vi "INI.vi"(0 "System no.":i32=1 min=1 max=4 step=1, 2 "INI axes":string[](array[string]), 3 "All axes?":bool, 4 "Axis identifier?":bool=TRUE, 5 "error in":errorcluster) -> (19 "error out":errorcluster)   [LabVIEW 2020]
doc: "Initializes axes. System-specific: see individual GCS-DLL or system manual for details.\n\nC-702: If All axes = TRUE, then Axis identifier must be TRUE\n\nC-843: If All axes = TRUE, then Axis identifier must be TRUE\n\nC-843.PM: If All axes = TRUE, then Axis identifier must be TRUE\n\nC-844: If All axes = TRUE, then Axis identifier must be TRUE, It is necessary to wait a certain time - appr. 4 s - before sending the next command to prevent it from being lost.\n\nC-848: If All axes = TRUE, then Axis identifier must be TRUE\n\nC-865: If All axes = TRUE, then Axis identifier must be TRUE\n\nC-866: If All axes? = TRUE, then Axis identifier? must be TRUE\n\nC-880: If All axes = TRUE, then Axis identifier must be TRUE\n\nC-885: All axes must beTRUE, Axis identifier must be FALSE\n\nE-710: If All axes = TRUE, then Axis identifier must be TRUE\n\nC-887, F-206, M-8X0: Only for GCS syntax version = GCS 1.0 (Check with CSV?.vi. If CSV?.vi is not supported, syntax version is GCS 1.0). For GCS 2.0 or higher, VI calls FRF instead for compatibility. To initialize hexapod, All axes = TRUE, Axis identifier = FALSE, (separate axes A,B (if present) will not be initialized); to initialize axes A,B: All axes = FALSE; VI will not wait for INI procedure to finish. Depending on the firmware version on the controller, motion initiated by INI may not be able to be stopped by STOP, #24 or #27.\n\nHydra, Pollux: If All axes? = TRUE, then Axis identifier? can be FALSE.\n\nMercury: If All axes = TRUE, then Axis identifier can be FALSE"
uses:
  Controller names.ctl
  Syntax.ctl
  Global2 (Array).vi
  Global1.vi
panel:
  # "Initializes axes. System-specific: see individual\nGCS-DLL or system manual for details."
  # "If all axes: use"
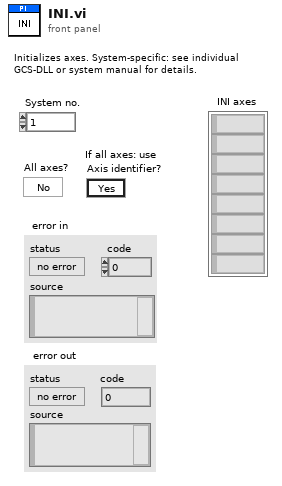
[diagram p1: front panel]
types:
  T1 = typedef "Syntax.ctl" = enum16{"GCS 1.0", "GCS 2.0", "GCS 3.0"}
  T2 = typedef "Controller names.ctl" = enum16{"None", "Analog", "C-702", "C-413", "C-414", "C-843", "C-843.PM", "C-844", "C-848", "C-865", "C-866", "C-867", "C-877", "C-880", "C-884", "C-885", "C-886", "C-887", "C-891", "E-135", "E-516", "E-517", "E-518", "E-709", "E-710", "E-712", "E-725", "E-727", "E-753", "E-754", "E-755", "E-761", "E-816", "E-861", "E-870", "E-871", "E-872", "E-873", "E-874", "F-206", "HydraPollux", "M-840", "M-850", "M-8X0", "Mercury", "Mercury_GCS", "PI_GCS2"}
  T3 = cluster{"Conn. axes":string[], "Controller name":T2}[]
  T4 = cluster{"Conn. axes":string[], "Controller name":T2}
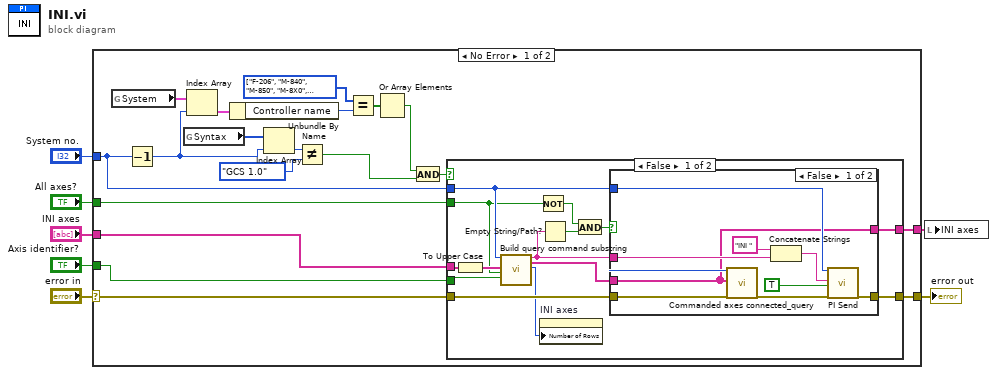
[diagram p0: block diagram]
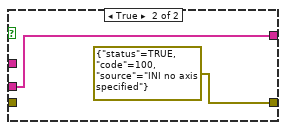
[diagram p2: hidden frame]
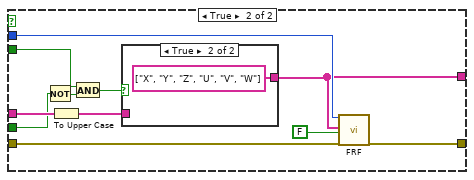
[diagram p3: hidden frame]
diagram:
  n1 = case shown="No Error" "error in" {
    selector: "error in" -> [w11 w66]
    tunnel: "INI axes" -> [w26 w65]
    tunnel: "Axis identifier?" -> [w25 _]
    tunnel: "System no." -> [w13 _]
    tunnel: "All axes?" -> [w24 _]
    tunnel: [w23 w66] -> w3
    tunnel: [w10 w65] -> w1
    frame No Error {
      w21 = T2[] [enum."F-206", enum."M-840", enum."M-850", enum."M-8X0", enum."C-887"] items=["None", "Analog", "C-702", "C-413", "C-414", "C-843", "C-843.PM", "C-844", "C-848", "C-865", "C-866", "C-867", "C-877", "C-880", "C-884", "C-885", "C-886", "C-887", "C-891", "E-135", "E-516", "E-517", "E-518", "E-709", "E-710", "E-712", "E-725", "E-727", "E-753", "E-754", "E-755", "E-761", "E-816", "E-861", "E-870", "E-871", "E-872", "E-873", "E-874", "F-206", "HydraPollux", "M-840", "M-850", "M-8X0", "Mercury", "Mercury_GCS", "PI_GCS2"]
      n2 = global read "Global2 (Array).vi" "System"() -> (w18:T3)
      n3 = Decrement(x=w13) -> (x-1=w9:i32)
      n4 = global read "Global1.vi" "Syntax"() -> (w17:T1[])
      n5 = Index Array(array=w18, index=w9) -> (element=w19:T4)
      n6 = Unbundle By Name(w19) -> ("Controller name"=w20:T2)
      n7 = Index Array(array=w17, index=w9) -> (element=w16:T1)
      n8 = Not Equal?(x=w16, y=Syntax."GCS 1.0") -> (x != y?=w15:bool)
      n9 = Equal?(x=w21, y=w20) -> (x = y?=w22:bool[])
      n10 = Or Array Elements(Boolean array=w22) -> (logical OR=w14:bool)
      n11 = And(x=w14, y=w15) -> (x .and. y?=w12:bool)
      n12 = case shown="False" w12 {
        tunnel: w11 -> [w40 w60]
        tunnel: w26 -> [w39 w62]
        tunnel: w25 -> [w37 w54]
        tunnel: w13 -> [w36 w61]
        tunnel: w24 -> [w34 w55]
        tunnel: [w32 w57] -> w23
        tunnel: [w31 w52] -> w10
        frame False {
          n13 = To Upper Case(1:w39) -> (0:w38:string[])
          n14 = call "Build query command substring.vi"("System no."=w36, "Axes to query in"=w38, "Query\nAll axes?"=w34, "For all axes: use\nAxis identifier?"=w37) -> ("Command substring"=w28:string, "Axes to query out"=w30:string[], "Number of rows"=w35:u32)  [unwired: 2 in, 11 out]
          n15 = Not(x=w34) -> (.not. x?=w33:bool)
          n16 = Empty String/Path?(string/path=w28) -> (empty?=w27:bool)
          n17 = property on="INI axes" class="Arr (strict)"("Number of Rows"=w35) -> ()  [unwired: 2 in, 2 out]
          n18 = And(x=w33, y=w27) -> (x .and. y?=w29:bool)
          n19 = case shown="False" w29 {
            tunnel: w40 -> [w46 _]
            tunnel: w28 -> [w45 _]
            tunnel: w36 -> [w44 _]
            tunnel: [w42 errorcluster {"status"=TRUE, "code"=100, "source"="INI no axis specified"} ("error out")] -> w32
            tunnel: [w41 w50] -> w31
            tunnel: w30 -> [w41 w50]
            frame False {
              n20 = call "Commanded axes connected_query.vi"("System no."=w44, "Commanded axes"=w41, "error in"=w46) -> ("error out"=w43:errorcluster)  [unwired: 1 in, 15 out]
              n21 = Concatenate Strings("INI ", w45) -> (w47:string)
              n22 = call "PI Send.vi"("System no."=w44, "String to send"=w47, "Attach termination char.?"=TRUE ("Attach Linefeed?"), "error in"=w43) -> ("error out"=w42:errorcluster)  [unwired: 2 in, 13 out]
            }
            frame True {
            }
          }
        }
        frame True {
          n23 = Not(x=w54) -> (.not. x?=w53:bool)
          n24 = To Upper Case(1:w62) -> (0:w58:string[])
          n25 = And(x=w55, y=w53) -> (x .and. y?=w56:bool)
          n26 = case shown="True" w56 {
            tunnel: w58 -> [w63 _]
            tunnel: [w63 string[] ["X", "Y", "Z", "U", "V", "W"] ("Conn. axes")] -> w52
            frame False {
            }
            frame True {
            }
          }
          n27 = call "FRF.vi"("System no."=w61, "Affected axes"=w52, "All axes?"=FALSE, "error in"=w60) -> ("error out"=w57:errorcluster)  [unwired: 1 in, 14 out]
        }
      }
    }
    frame Error {
    }
  }
  "error out" <- w3
  n28 = local write "INI axes"(w1) -> ()
